vi "Datalogger Path--constant.vi"(8 "Error In":errorcluster) -> (0 "Error Out":errorcluster, 3 "Path":path)   [LabVIEW 2024, in "UIs Handler.lvlib"]
uses:
  UIs Handler.lvlib
  <userlib>/_MGI/File/MGI Create Directory Chain Behavior Enum.ctl
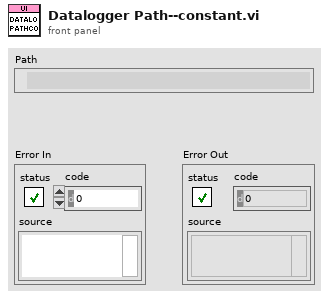
[diagram p1: front panel]
types:
  T1 = typedef "MGI Create Directory Chain Behavior Enum.ctl" = enum16{"Auto Detect", "Path Contains a File", "Path Does Not Contain a File"}
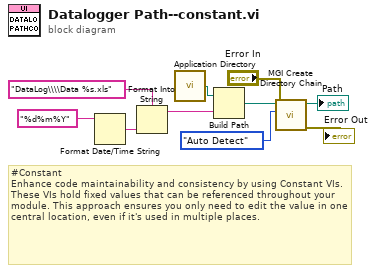
[diagram p0: block diagram]
diagram:
  # "#Constant\nEnhance code maintainability and consistency by using Constant VIs. These VIs hold fixed values that can be referenced throughout your module. This approach ensures you only need to edit the value in one central location, even if it's used in multiple places."
  n1 = Format Date/Time String(time format string (%c)="%d%m%Y") -> (date/time string=w6:string)  [unwired: 2 in]
  n2 = Format Into String(format string="DataLog\\\\Data %s.xls", w6) -> (resulting string=w5:string)  [unwired: 2 in, 1 out]
  n3 = call <vilib>:"Application Directory.vi"() -> ("Application Directory"=w9:path)
  n4 = Build Path(base path=w9, name or relative path=w5) -> (appended path=w8:path)
  n5 = call <userlib>:"MGI Create Directory Chain.vi"("Error In"="Error In", "File Presence (Auto Detect)"=MGI_Create_Directory_Chain_Behavior_Enum."Auto Detect", "Path"=w8) -> ("Error Out"=→"Error Out":errorcluster, "Duplicate Path"=→"Path":path)  [unwired: 7 in]
